vi "LED_Circuit.vi"() -> ()   [LabVIEW 2023]
panel:
  in  "stop":bool
  in  "VISA resource name 2":refnum<visa-resource-name>
  out "Numeric":dbl
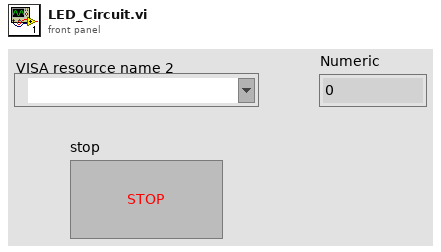
[diagram p1: front panel]
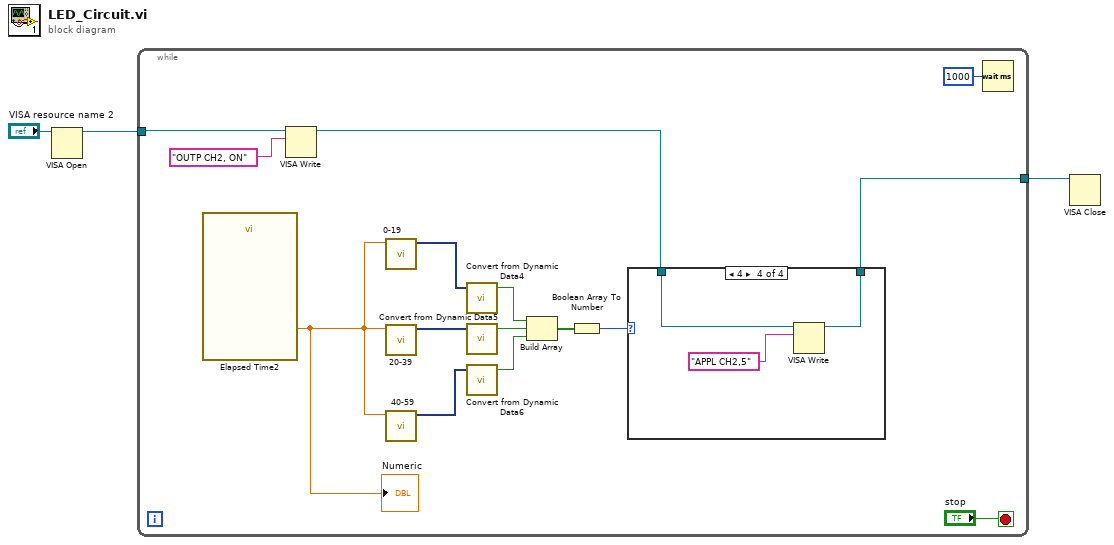
[diagram p0: block diagram]
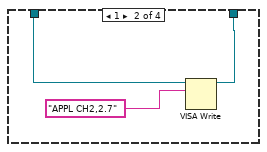
[diagram p3: hidden frame]
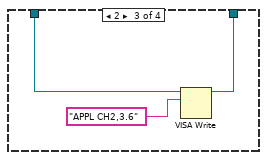
[diagram p4: hidden frame]
diagram:
  n1 = VISA Open(VISA resource name="VISA resource name 2") -> (VISA resource name=w3:refnum<visa-resource-name>)  [unwired: 4 in, 1 out]
  n2 = while {
    tunnel: w3 -> [w9]
    tunnel: [w7] -> w1
    stop <- "stop" stop-if-true
    n3 = call "Elapsed Time2"() -> ("Elapsed Time (s)"=w4:dbl)  [unwired: 12 in, 7 out]
    "Numeric" <- w4
    n4 = VISA Write(VISA resource name=w9, write buffer="OUTP CH2, ON") -> (VISA resource name out=w10:refnum<visa-resource-name>)  [unwired: 1 in, 2 out]
    n5 = call "0-19"("Operand 1"=w4) -> ("Result"=w18:dynamicdata)  [unwired: 9 in, 1 out]
    n6 = call "20-39"("Operand 1"=w4) -> ("Result"=w17:dynamicdata)  [unwired: 9 in, 1 out]
    n7 = call "40-59"("Operand 1"=w4) -> ("Result"=w16:dynamicdata)  [unwired: 9 in, 1 out]
    n8 = call "Convert from Dynamic Data4"("Dynamic Data Type"=w18) -> ("Scalar"=w14:bool)  [unwired: 3 in]
    n9 = call "Convert from Dynamic Data5"("Dynamic Data Type"=w17) -> ("Scalar"=w15:bool)  [unwired: 3 in]
    n10 = call "Convert from Dynamic Data6"("Dynamic Data Type"=w16) -> ("Scalar"=w13:bool)  [unwired: 3 in]
    n11 = Build Array(w14, w15, w13) -> (w12:bool[])
    n12 = Boolean Array To Number(Boolean array=w12) -> (number=w11:u32)
    n13 = case shown="4" w11 {
      tunnel: w10 -> [w19 w22 w24 w26]
      tunnel: [w19 w21 w23 w27] -> w7
      frame 0, Default {
      }
      frame 1 {
        n14 = VISA Write(VISA resource name=w22, write buffer="APPL CH2,2.7") -> (VISA resource name out=w21:refnum<visa-resource-name>)  [unwired: 1 in, 2 out]
      }
      frame 2 {
        n15 = VISA Write(VISA resource name=w24, write buffer="APPL CH2,3.6") -> (VISA resource name out=w23:refnum<visa-resource-name>)  [unwired: 1 in, 2 out]
      }
      frame 4 {
        n16 = VISA Write(VISA resource name=w26, write buffer="APPL CH2,5") -> (VISA resource name out=w27:refnum<visa-resource-name>)  [unwired: 1 in, 2 out]
      }
    }
    n17 = Wait (ms)(milliseconds to wait=u32 1000) -> ()  [unwired: 1 out]
  }
  n18 = VISA Close(VISA resource name=w1) -> ()  [unwired: 1 in, 1 out]
